vi "MicroPulse - uptime msg assembly.vi"(9 "SRST":u32, 10 "RST":u32, 11 "Uptime":u32) -> (3 "String":string)   [LabVIEW 2026, in "MicroPulse_Driver.lvlib"]
uses:
  MicroPulse_Driver.lvlib
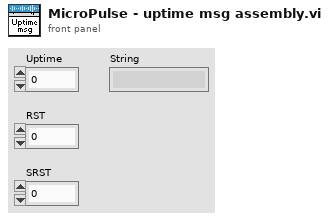
[diagram p1: front panel]
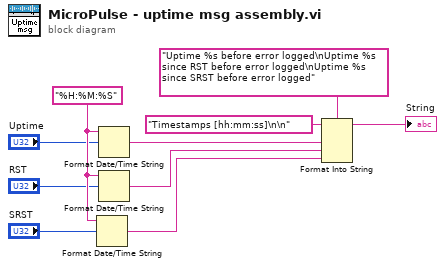
[diagram p0: block diagram]
diagram:
  w7 = "%H:%M:%S" ("time format string (%c)")
  n1 = Format Date/Time String(time format string (%c)=w7, seconds (now)="SRST") -> (date/time string=w9:string)  [unwired: 1 in]
  n2 = Format Date/Time String(time format string (%c)=w7, seconds (now)="Uptime") -> (date/time string=w4:string)  [unwired: 1 in]
  n3 = Format Date/Time String(time format string (%c)=w7, seconds (now)="RST") -> (date/time string=w8:string)  [unwired: 1 in]
  n4 = Format Into String(format string="Uptime %s before error logged\nUptime %s since RST before error logged\nUptime %s since SRST before error logged", initial string="Timestamps [hh:mm:ss]\n\n", w4, w8, w9) -> (resulting string=→"String":string)  [unwired: 1 in, 1 out]
